vi "Write visa resource name.vi"(8 "error in (no error)":errorcluster, 10 "visa resource name":refnum<visa-resource-name>, 11 "ELAN Data Unit in":refnum<class "ELAN Data Unit.lvclass">) -> (0 "error out":errorcluster, 3 "ELAN Data Unit out":refnum<class "ELAN Data Unit.lvclass">)   [LabVIEW 2021, in "ELAN Data Unit.lvclass"]
uses:
  ELAN Data Unit.lvclass
  ELAN Data Unit.lvclass/ELAN Data Unit.ctl
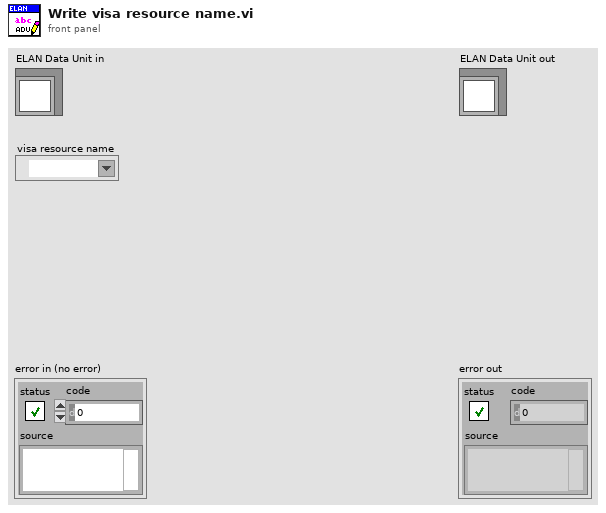
[diagram p1: front panel]
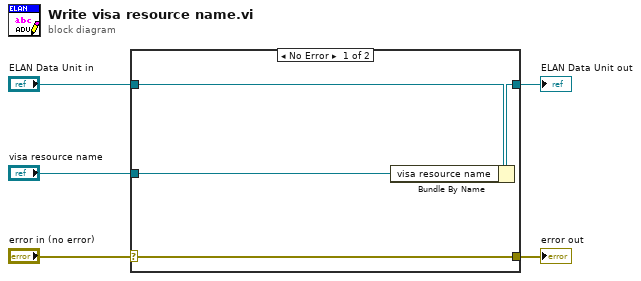
[diagram p0: block diagram]
diagram:
  n1 = case shown="No Error" "error in (no error)" {
    selector: "error in (no error)" -> [w9 w10]
    tunnel: [w9 w10] -> w4
    tunnel: [w7 w11] -> w2
    tunnel: "ELAN Data Unit in" -> [w8 w11]
    tunnel: "visa resource name" -> [w6 _]
    frame No Error {
      n2 = Bundle By Name(cluster=w8, "visa resource name"=w6) -> (w7:refnum<class "ELAN Data Unit.lvclass">)
    }
    frame Error {
    }
  }
  "error out" <- w4
  "ELAN Data Unit out" <- w2
